vi "InterruptMove.vi"(6 "error in":errorcluster, 9 "VISA resource In":refnum<visa-resource-name>) -> (0 "error out":errorcluster, 3 "VISA resource name out":refnum<visa-resource-name>)   [LabVIEW 2016]
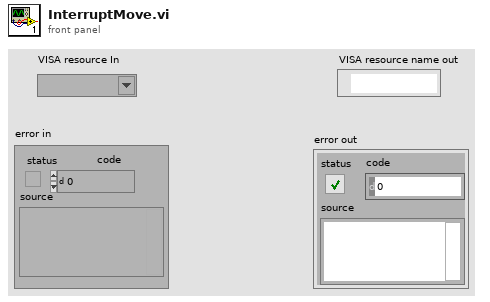
[diagram p1: front panel]
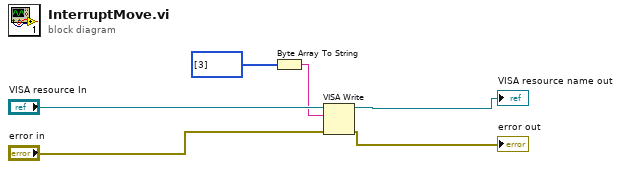
[diagram p0: block diagram]
diagram:
  n1 = Byte Array To String(unsigned byte array=u8[] [3]) -> (string=w3:string)
  n2 = VISA Write(VISA resource name="VISA resource In", write buffer=w3, error in (no error)="error in") -> (VISA resource name out=→"VISA resource name out":refnum<visa-resource-name>, error out=→"error out":errorcluster)  [unwired: 1 out]
